vi "Destroy.vi"(8 "Error In":errorcluster, 11 "Context":refnum<class "Context.lvclass">) -> (0 "Error Out":errorcluster, 2 "Hooks":T1)   [LabVIEW 2018, in "Toolkit.lvlib" / "Context.lvclass"]
doc: "Safely destroys a Context object and frees any internal resources. Once a Context object is destroyed it cannot be used."
uses:
  Context.lvclass
  Type Definitions/Hooks.ctl
  Hooks/Render/Render/Process.lvclass
  Hooks/Render/Section/Section.lvclass
  Hooks/Render/Variable/Variable.lvclass
  Context.lvclass/Context.ctl
  Toolkit.lvlib
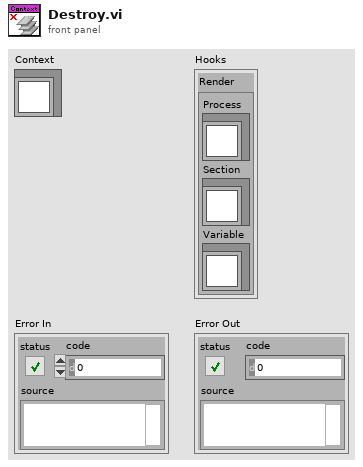
[diagram p1: front panel]
types:
  T1 = typedef "Toolkit.lvlib/Hooks.ctl" = cluster{"Render":cluster{"Process":refnum<class "Process.lvclass">, "Section":refnum<class "Section.lvclass">, "Variable":refnum<class "Variable.lvclass">}}
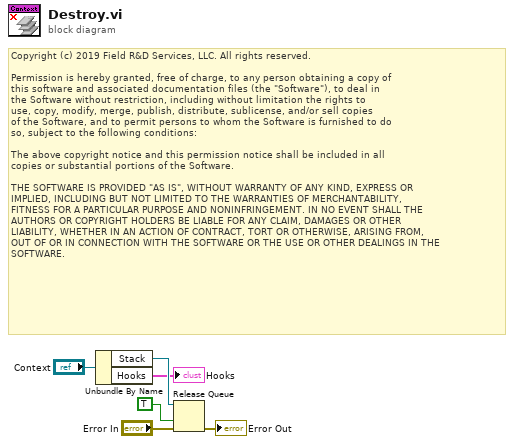
[diagram p0: block diagram]
diagram:
  # "Copyright (c) 2019 Field R&D Services, LLC. All rights reserved.\n\nPermission is hereby granted, free of charge, to any person obtaining a copy of\nthis software and associated documentation files (the \"Software\"), to deal in\nthe Software without restriction, including without limitation the rights to\nuse, copy, modify, merge, publish, distribute, sublicense, and/or sell copies\nof the Software, and to permit persons to whom the Software is furnished to do\nso, subject to the following conditions:\n\nThe above copyright notice and this permission notice shall be included in all\ncopies or substantial portions of the Software.\n\nTHE SOFTWARE IS PROVIDED \"AS IS\", WITHOUT WARRANTY OF ANY KIND, EXPRESS OR\nIMPLIED, INCLUDING BUT NOT LIMITED TO THE WARRANTIES OF MERCHANTABILITY,\nFITNESS FOR A PARTICULAR PURPOSE AND NONINFRINGEMENT. IN NO EVENT SHALL THE\nAUTHORS OR COPYRIGHT HOLDERS BE LIABLE FOR ANY CLAIM, DAMAGES OR OTHER\nLIABILITY, WHETHER IN AN ACTION OF CONTRACT, TORT OR OTHERWISE, ARISING FROM,\nOUT OF OR IN CONNECTION WITH THE SOFTWARE OR THE USE OR OTHER DEALINGS IN THE\nSOFTWARE."
  n1 = Unbundle By Name("Context") -> ("Stack"=w5:refnum<queue>, "Hooks"=→"Hooks":T1)
  n2 = Release Queue(queue=w5, force destroy? (F)=TRUE, error in (no error)="Error In") -> (error out=→"Error Out":errorcluster)  [unwired: 2 out]
